vi "Connect Sequence View.vi"(8 "error in (no error)":errorcluster, 11 "teststand-api in":refnum<class "teststand-api.lvclass">) -> (0 "error out":errorcluster, 3 "teststand-api out":refnum<class "teststand-api.lvclass">)   [LabVIEW 2014, in "teststand-api.lvlib" / "teststand-api.lvclass"]
uses:
  teststand-api.lvclass
  teststand-api.lvclass/teststand-api.ctl
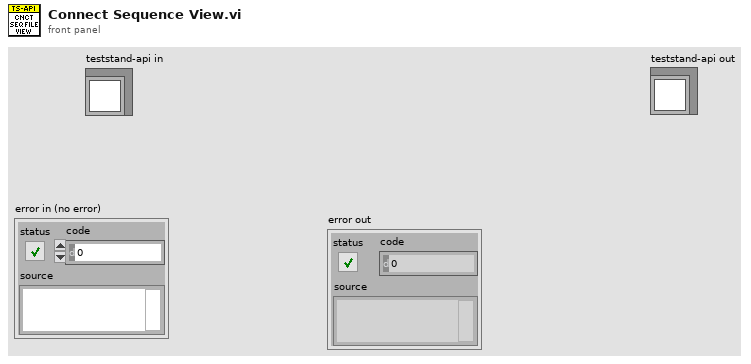
[diagram p1: front panel]
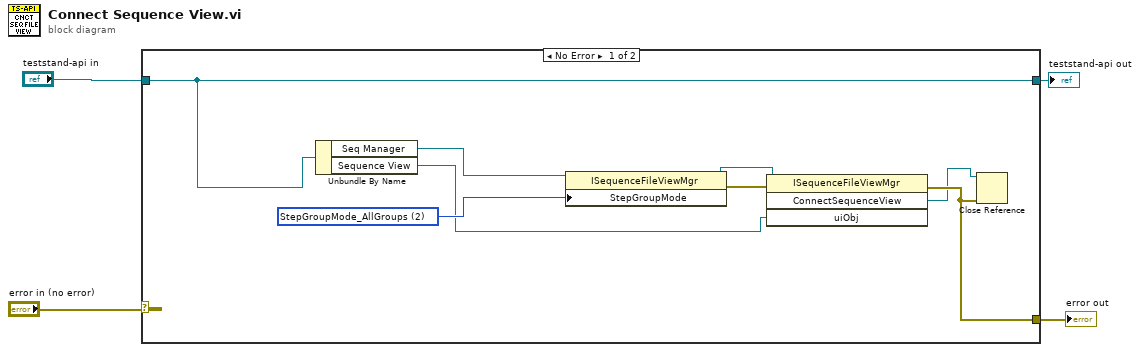
[diagram p0: block diagram]
diagram:
  n1 = case shown="No Error" "error in (no error)" {
    selector: "error in (no error)" -> [_ w14]
    tunnel: [w12 w14] -> w3
    tunnel: "teststand-api in" -> [w5 w13]
    tunnel: [w5 w13] -> w1
    frame No Error {
      w9 = 2 items=["StepGroupMode_OneGroup"=1, "StepGroupMode_AllGroups"=2] ("StepGroupMode")
      n2 = Unbundle By Name(w5) -> ("Seq Manager"=w8:refnum<k7>, "Sequence View"=w7:refnum<k7>)
      n3 = property class="ISequenceFileViewMgr"(reference=w8, "StepGroupMode"=w9) -> (reference out=w11:refnum<k7>, error out=w10:errorcluster)  [unwired: 1 in]
      n4 = invoke class="ISequenceFileViewMgr" method="ConnectSequenceView"(reference=w11, error in=w10, "uiObj"=w7) -> (error out=w12:errorcluster, "ConnectSequenceView"=w6:refnum<k7>)  [unwired: 1 in, 2 out]
      n5 = Close Reference(reference=w6, error in (no error)=w12) -> ()  [unwired: 1 out]
    }
    frame Error {
    }
  }
  "error out" <- w3
  "teststand-api out" <- w1
